vi "3 Position Switch.vi"(1 "Downward Direction":bool, 2 "Upward Direction":bool) -> (0 "3 Position Switch (0 = Down, 1 = Middle, 2 = Up)":dbl)   [LabVIEW 2014]
doc: "This VI converts two boolean inputs (assumed to be from the control board) into a number that describes the location of the three position switch. The operational assumption is that if both the upward direction and downward direction booleans are either true or false, the switch is in the neutral (or middle) position. If the downward direction boolean is true, and the upward is false, the switch is in the down position. If the downward direction is false, and the upward is true, the switch is in the up position"
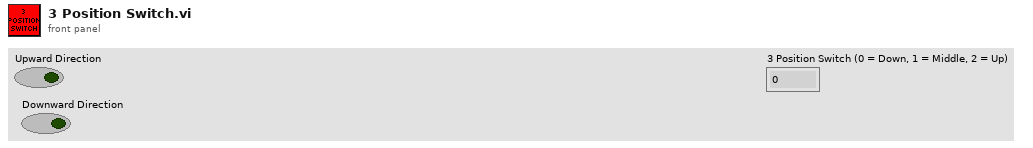
[diagram p1: front panel]
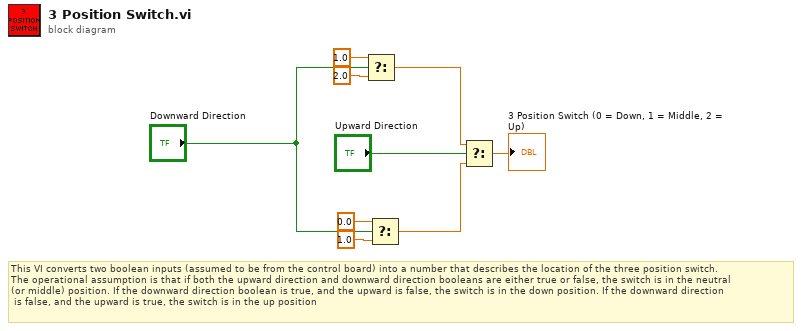
[diagram p0: block diagram]
diagram:
  # "This VI converts two boolean inputs (assumed to be from the control board) into a number that describes the location of the three position switch. \nThe operational assumption is that if both the upward direction and downward direction booleans are either true or false, the switch is in the neutral \n(or middle) position. If the downward direction boolean is true, and the upward is false, the switch is in the down position. If the downward direction\n is false, and the upward is true, the switch is in the up position"
  n1 = Select(t=1.0, s="Downward Direction", f=2.0) -> (s? t:f=w3:dbl)
  n2 = Select(t=0.0, s="Downward Direction", f=1.0) -> (s? t:f=w9:dbl)
  n3 = Select(t=w3, s="Upward Direction", f=w9) -> (s? t:f=→"3 Position Switch (0 = Down, 1 = Middle, 2 = Up)":dbl)
